vi "DynamicEvent.vi"() -> ()   [LabVIEW 2012]
panel:
  in  "Stop":bool
  in  "IncValue":i32
  in  "Increment":bool
  out "Stop":i32
  out "Timeout":i32
  out "Count":i32
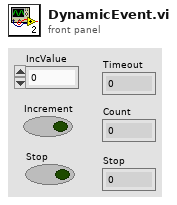
[diagram p1: front panel]
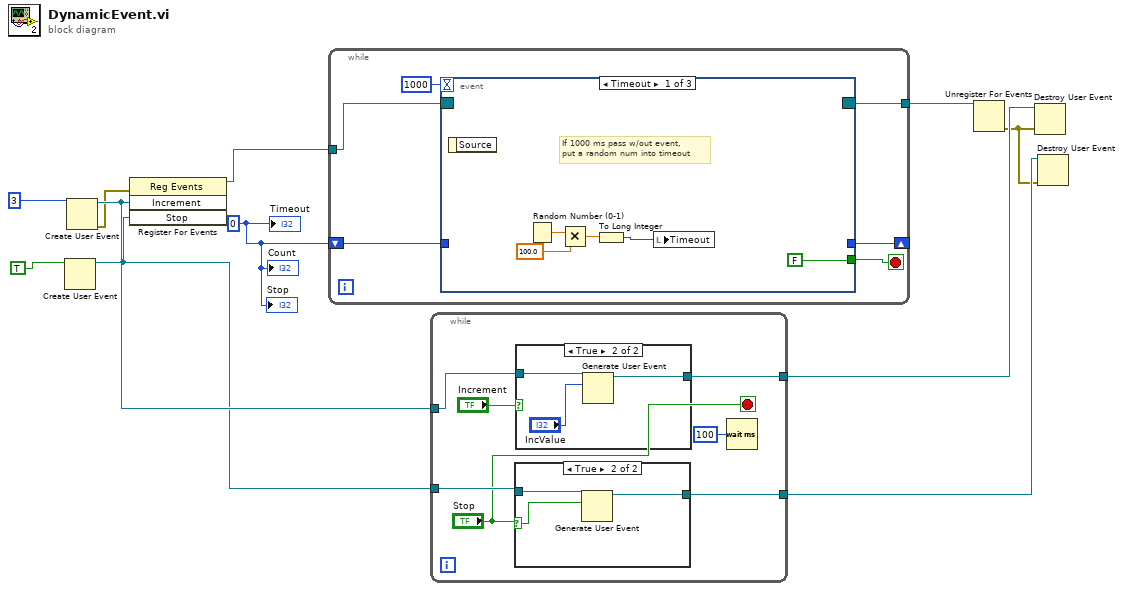
[diagram p0: block diagram]
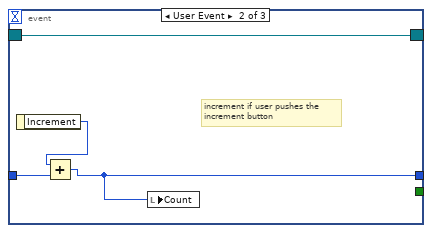
[diagram p4: hidden frame]
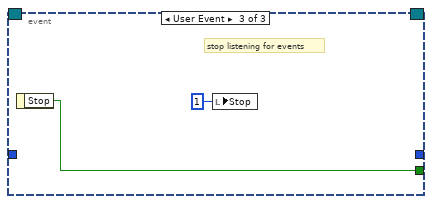
[diagram p5: hidden frame]
diagram:
  w11 = 0 ("Timeout")
  n1 = Create User Event(user event datatype=TRUE ("Stop")) -> (user event=w3:refnum<user-event>)  [unwired: 1 in, 1 out]
  n2 = Create User Event(user event datatype=3 ("Increment")) -> (user event=w7:refnum<user-event>, error out=w5:errorcluster)  [unwired: 1 in]
  n3 = register-events(error in=w5, w7, w3) -> (reference out=w9:refnum<event-registration>)  [unwired: 1 in, 1 out]
  n4 = while {
    shift-right: [w13] -> _
    shift-left: w11 -> [w14]
    tunnel: w9 -> [w15]
    tunnel: [w12] -> w8
    stop <- w16 stop-if-true
    n5 = event shown="[0] Timeout" {
      selector: w15 -> [_ w23 _]
      dyn-events: [_ w23 _] -> w12
      timeout: 1000 -> [_ _ _]
      tunnel: [FALSE _ w28] -> w16
      tunnel: w14 -> [_ w26 _]
      tunnel: [_ w24 _] -> w13
      event Timeout {
        # "If 1000 ms pass w/out event,\nput a random num into timeout"
        n6 = event-data() -> ()  [unwired: 1 in, 1 out]
        n7 = Random Number (0-1)() -> (number: 0 to 1=w21:dbl)
        n8 = Multiply(x=w21, y=100.0) -> (x*y=w19:dbl)
        n9 = To Long Integer(number=w19) -> (32bit integer=w18:i32)
        n10 = local write "Timeout"(w18) -> ()
      }
      event User Event {
        # "increment if user pushes the\nincrement button"
        n11 = event-data() -> ("Increment"=w25:i32)  [unwired: 1 in]
        n12 = Add(x=w25, y=w26) -> (x+y=w24:i32)
        n13 = local write "Count"(w24) -> ()
      }
      event User Event {
        # "stop listening for events"
        n14 = event-data() -> ("Stop"=w28:bool)  [unwired: 1 in]
        n15 = local write "Stop"(1 ("Stop")) -> ()
      }
    }
  }
  n16 = while {
    tunnel: w7 -> [w33]
    tunnel: [w32] -> w6
    tunnel: w3 -> [w31]
    tunnel: [w30] -> w2
    stop <- "Stop" stop-if-true
    n17 = case shown="True" "Stop" {
      selector: "Stop" -> [_ w37]
      tunnel: w31 -> [w36 w39]
      tunnel: [w36 w38] -> w30
      frame False {
      }
      frame True {
        n18 = Generate User Event(user event=w39, event data cluster=w37) -> (user event out=w38:refnum<user-event>)  [unwired: 1 in, 1 out]
      }
    }
    n19 = case shown="True" "Increment" {
      tunnel: w33 -> [w40 w43]
      tunnel: [w40 w42] -> w32
      frame False {
      }
      frame True {
        n20 = Generate User Event(user event=w43, event data cluster="IncValue") -> (user event out=w42:refnum<user-event>)  [unwired: 1 in, 1 out]
      }
    }
    n21 = Wait (ms)(milliseconds to wait=u32 100) -> ()  [unwired: 1 out]
  }
  n22 = Unregister For Events(event registration refnum=w8) -> (error out=w1:errorcluster)  [unwired: 1 in]
  n23 = Destroy User Event(user event=w6, error in=w1) -> ()  [unwired: 1 out]
  n24 = Destroy User Event(user event=w2, error in=w1) -> ()  [unwired: 1 out]
  "Count" <- w11
  "Timeout" <- w11
  "Stop" <- w11
